vi "RX Message.vi"(8 "error in (no error)":errorcluster, 11 "Engine RPM in":refnum<class "Engine RPM.lvclass">) -> (0 "error out":errorcluster, 2 "String":string, 3 "Engine RPM out":refnum<class "Engine RPM.lvclass">)   [LabVIEW 2011, in "Engine RPM.lvclass"]
uses:
  Engine RPM.lvclass
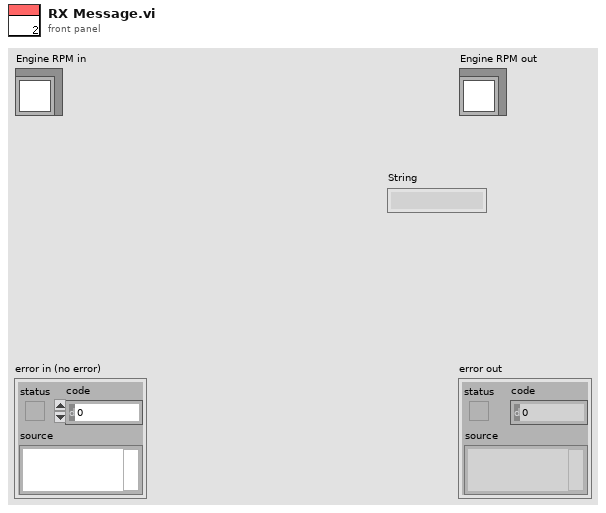
[diagram p1: front panel]
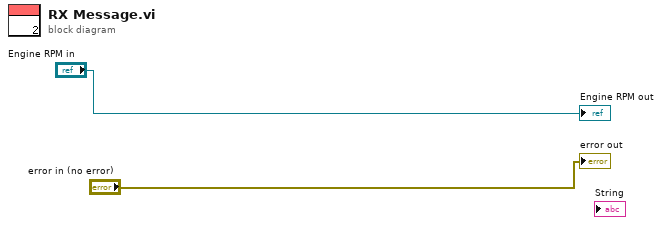
[diagram p0: block diagram]
diagram:
  "error out" <- "error in (no error)"
  "Engine RPM out" <- "Engine RPM in"
